vi "Helmholtz2D_Cal RHS.vi"(8 "Boundary Condition":cluster{"type":T1, "Value":dbl[]}[](array[cluster]) {"type" items=["Dirichlet", "Neumann"]}, 9 "Domain":T2={"x"={"start x"=0.0, "end x"=1.0, "# of x-points"=11}, "y"={"start y"=0.0, "end y"=1.0, "# of y-points"=11}}, 10 "k":dbl=1.0, 11 "F(x, y)":dbl[][](array[numeric])) -> (3 "RHS":dbl[](array[numeric]))   [LabVIEW 2020, in "NI_PDE.lvlib"]
uses:
  <vilib>/gmath/NI_PDE.lvlib
  <vilib>/gmath/pde.llb/Common/PDE_BC Type.ctl
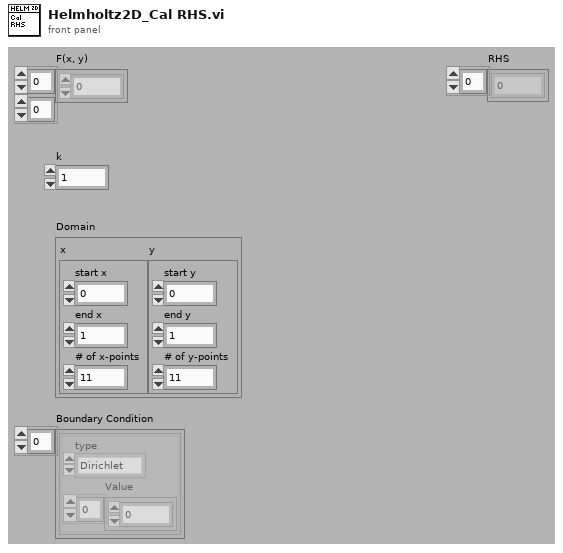
[diagram p1: front panel]
types:
  T1 = typedef "NI_PDE.lvlib/PDE_BC Type.ctl" = i32
  T2 = cluster{"x":cluster{"start x":dbl, "end x":dbl, "# of x-points":i32}, "y":cluster{"start y":dbl, "end y":dbl, "# of y-points":i32}}
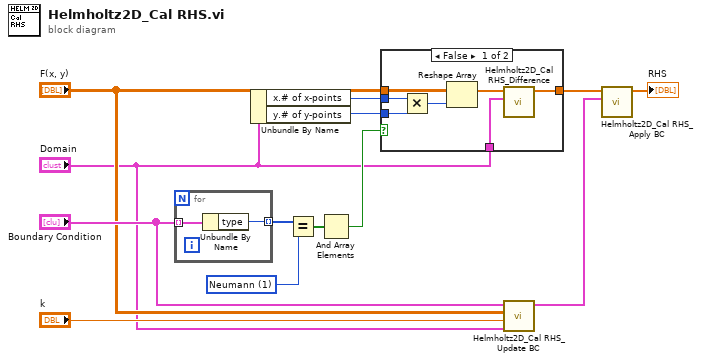
[diagram p0: block diagram]
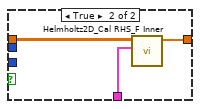
[diagram p2: hidden frame]
diagram:
  w12 = T1 1 items=["Dirichlet", "Neumann"] ("type")
  n1 = for {
    tunnel: "Boundary Condition" -> [w15] mode=indexing
    tunnel: [w14] -> w13 mode=indexing
    n2 = Unbundle By Name(w15) -> ("type"=w14:T1)
  }
  n3 = Unbundle By Name("Domain") -> ("x.# of x-points"=w9:i32, "y.# of y-points"=w8:i32)
  n4 = Equal?(x=w13, y=w12) -> (x = y?=w11:bool[])
  n5 = And Array Elements(Boolean array=w11) -> (logical AND=w10:bool)
  n6 = case shown="False" w10 {
    tunnel: "F(x, y)" -> [w22 w25]
    tunnel: "Domain" -> [w20 w24]
    tunnel: w9 -> [w18 _]
    tunnel: w8 -> [w17 _]
    tunnel: [w16 w23] -> w2
    frame False {
      n7 = Multiply(x=w18, y=w17) -> (x*y=w19:i32)
      n8 = Reshape Array(w22, w19) -> (w21:dbl[])
      n9 = call <vilib>:"Helmholtz2D_Cal RHS_Difference.vi"("Domain"=w20, "X"=w21) -> ("Diff X"=w16:dbl[])  [unwired: 9 out]
    }
    frame True {
      n10 = call <vilib>:"Helmholtz2D_Cal RHS_F Inner.vi"("Domain"=w24, "F(x, y)"=w25) -> ("F Inner"=w23:dbl[])  [unwired: 9 out]
    }
  }
  n11 = call <vilib>:"Helmholtz2D_Cal RHS_Update BC.vi"("Domain"="Domain", "k"="k", "F(x, y)"="F(x, y)", "Boundary Condition In"="Boundary Condition") -> ("Boundary Condition Out"=w3:cluster{"type":T1, "Value":dbl[]}[])  [unwired: 7 out]
  n12 = call <vilib>:"Helmholtz2D_Cal RHS_Apply BC.vi"("Boundary Condition"=w3, "RHS In"=w2) -> ("RHS Out"=→"RHS":dbl[])  [unwired: 9 out]
